vi "Problema1_2.vi"() -> ()   [LabVIEW 2020]
panel:
  in  "String":string
  out "String":string
  out "Thermometer":dbl(slide) scale=0.0..100.0
  in  "DBL":dbl(knob) scale=0.0..100.0
  out "boleano 2":bool
  out "INT 2":i32
  in  "INT":i32
  in  "boleano":bool
  # "Funcionamiento"
  # "Controles para tipos de datos basicos(INT, DBL, Boolean, String)."
  # "INT: En este control se introduce un numero entero y se muestra en la otra casilla."
  # "DBL: Para este control se utilizo una perilla para regular la temperatura y se puede observar de una mejor forma en el termometro"
  # "Boolean: Para este control solo se muestran 2 estados, los cuales pueden ser true o falce."
  # "String: En este control se muestran las palabras escritas en el primer string"
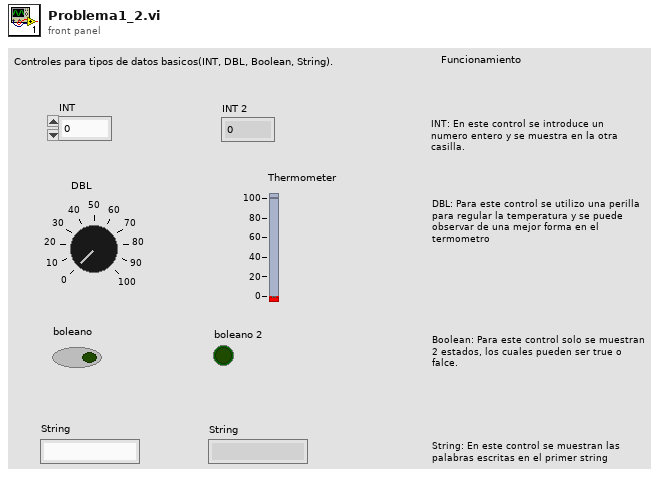
[diagram p1: front panel]
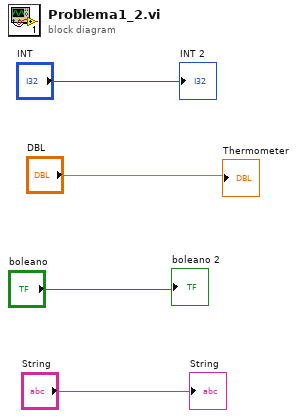
[diagram p0: block diagram]
diagram:
  "INT 2" <- "INT"
  "boleano 2" <- "boleano"
  "Thermometer" <- "DBL"
  "String" <- "String"
